vi "HardwareConfiguration.vi"() -> (3 "configured?":bool)   [LabVIEW 2013]
uses:
  InstrControl/InstrumentSetup.vi
  globals/QC_RunInformation.vi
  InstrControl/InstrControl.lvclass
panel:
  in  "Matrix Configurations":bool
  in  "Defaults Multimeter":bool
  in  "Multimeter":enum32{"Keithley 2000"}(tab)
  in  "Range Value\n(0.1 - 100)":dbl=100.0 format="%#.2g"
  in  "Range":u16(ring) items=["Auto", "Manual"]
  in  "Function":u16(ring)=3 items=["AC Current", "DC Current", "AC Voltage", "DC Voltage", "2W-Resistance", "4W-Resistance", "Period", "Frequency", "Temperature", "Diode", "Continuity"]
  in  "Address KE2000":refnum<visa-resource-name>
  in  "Defaults LCR":bool
  in  "LCRs":enum32{"WayneKerr 6440B", "WayneKerr 6425"}(tab)
  in  "AC frequency [Hz]":i32=1000 format="%#.3p"
  in  "RC Configuration":u16(ring) items=["serial", "parallel"]
  in  "AC amplitude [V]":sgl=0.1
  in  "Address WK6440B":refnum<visa-resource-name>
  in  "Address WK6425":refnum<visa-resource-name>
  in  "AC amplitude [V] WK6425":sgl=0.1 caption="AC amplitude [V]"
  in  "RC Configuration WK6425":u16(ring) caption="RC Configuration" items=["serial", "parallel"]
  in  "AC frequency [Hz] WK6425":i32=1000 caption="AC frequency [Hz]" format="%#.3p"
  in  "VISA address":refnum<visa-resource-name>="COM24" caption="Arduino address"
  out "Programm uploaded?":string="Make sure programme is uploaded to Arduino Uno ->"
  in  "Blank Button":bool
  in  "Supplies":T1(tab)
  in  "Front/Rear Output KE2410":u16(ring) caption="Front/Rear Output (not yet implemented)" items=["Front", "Rear"]
  in  "Current Limit [µA] 2410":sgl=100.0 caption="Current Limit [µA]"
  in  "Address KE2410":refnum<visa-resource-name>
  in  "Address KE2410_2":refnum<visa-resource-name>
  in  "Current Limit [µA] 2410_2":sgl=100.0 caption="Current Limit [µA]"
  in  "Front/Rear Output KE2410_2":u16(ring) caption="Front/Rear Output (not yet implemented)" items=["Front", "Rear"]
  in  "Address KE487":refnum<visa-resource-name>
  in  "Compliance":u16(ring) items=["20µA", "2mA"]
  in  "Range:":u16(ring) items=["Autorange", "2nA", "20nA", "200nA", "2 microAmp", "20 microAmp", "200 microAmp", "2 milliAmp"]
  in  "Current Limit 6517":u16(ring)=1 caption="Current Limit" items=["OFF", "ON"]
  in  "Address KE6517":refnum<visa-resource-name>
  in  "Address KE6517_2":refnum<visa-resource-name>
  in  "Current Limit 6517_2":u16(ring)=1 caption="Current Limit" items=["OFF", "ON"]
  in  "current compliance \nlevel [mA]":dbl=0.0001 format="%.4f"
  in  "compliance/measurement\nrange (auto:0)":u16(ring)=6 items=["auto / auto", "1 nA / 1.1 V", "10 nA / 11 V", "100 nA / 110 V", "0.001 mA / 110 V", "0.01 mA / 110 V", "0.1 mA / 110 V", "1 mA / 110 V", "10 mA / 110 V", "100 mA / 110 V"]
  in  "Address KE236":refnum<visa-resource-name>
  in  "Defaults Supply":bool
  in  "OK Button":bool
  # "Hardware Configuration"
  # "Multimeter Configuration"
  # "Supply Configuration"
  # "Arduino Configuration"
  # "LCR Configuration"
  # "(Only for initialisation)"
  # "(Only for initialisation)"
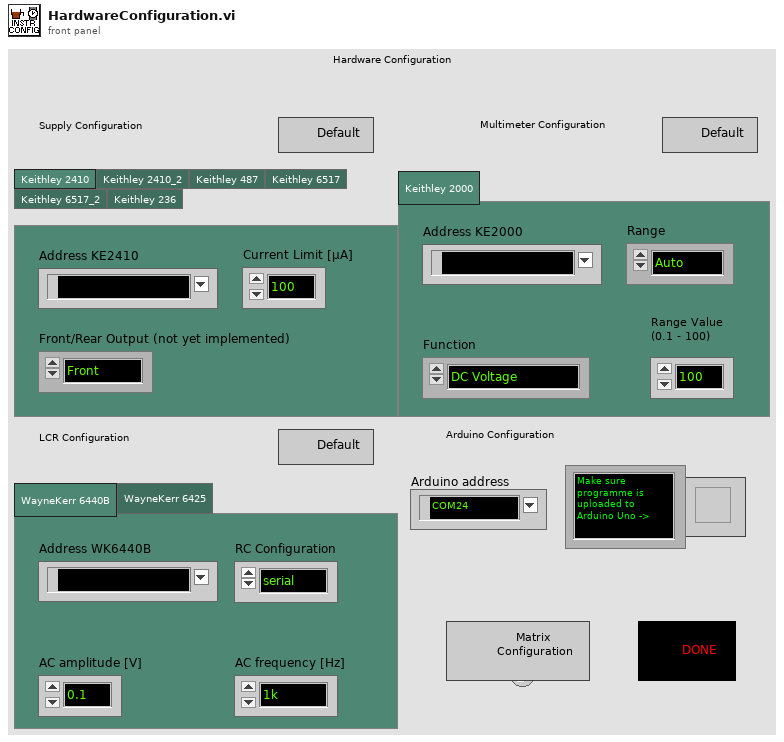
[diagram p1: front panel]
types:
  T1 = enum32{"Keithley 2410", "Keithley 2410_2", "Keithley 487", "Keithley 6517", "Keithley 6517_2", "Keithley 236"}
  T2 = cluster{"KE 2410":cluster{"Instrument name":string, "address":refnum<visa-resource-name>, "Instrument type":u16}, "KE 2410_2":cluster{"Instrument name":string, "address":refnum<visa-resource-name>, "Instrument type":u16}, "KE 6517":cluster{"Instrument name":string, "address":refnum<visa-resource-name>, "Instrument type":u16}, "KE 6517_2":cluster{"Instrument name":string, "address":refnum<visa-resource-name>, "Instrument type":u16}, "KE 487":cluster{"Instrument name":string, "address":refnum<visa-resource-name>, "Instrument type":u16}, "KE 236":cluster{"Instrument name":string, "address":refnum<visa-resource-name>, "Instrument type":u16}, "WK 6440B":cluster{"Instrument name":string, "address":refnum<visa-resource-name>, "Instrument type":u16}, "WK 6425":cluster{"Instrument name":string, "address":refnum<visa-resource-name>, "Instrument type":u16}, "HP 4263B":cluster{"Instrument name":string, "address":refnum<visa-resource-name>, "Instrument type":u16}, "Pickering Matrix":cluster{"Instrument name":string, "address":refnum<visa-resource-name>, "Instrument type":u16}, "KE 2000":cluster{"Instrument name":string, "address":refnum<visa-resource-name>, "Instrument type":u16}, "KE3706A Switching":cluster{"Instrument name":string, "address":refnum<visa-resource-name>, "Instrument type":u16}}
  T3 = cluster{"VISA address":refnum<visa-resource-name>, "T sensor":enum16{"SHT", "DS"}, "Arduino":refnum<class "ArduinoControl.lvclass">}
  T4 = cluster{"Range":u16, "Range Value":dbl, "Function":u16, "KE2000":refnum<class "KE2000.lvclass">}
  T5 = cluster{"Current Limit":sgl, "Front/Rear Output:":u16, "KE2410":refnum<class "KE2410.lvclass">}
  T6 = cluster{"Compliance":u16, "Range:":u16, "KE487":refnum<class "KE487.lvclass">}
  T7 = cluster{"Current Limit":u16, "KE6517":refnum<class "KE6517.lvclass">}
  T8 = cluster{"current \ncompliance level":dbl, "compliance/\nmeasurement range (auto:0)":u16, "KE236":refnum<class "KE236.lvclass">}
  T9 = cluster{"Sensor Serial No.:":string, "Wafer:":string, "Batch:":string, "Manufacturer:":string, "Device Category:":string, "Database Serial No.:":string, "Date Initiated:":string, "Time Initiated:":string, "Test":string, "Probeplan used:":string, "End of Run comment:":string, "User:":string, "Vbias SMU":string, "LCR":string, "Test SMU":string, "Test DMM":string}
  T10 = cluster{"RC Configuration":u16, "AC amplitude [V]":dbl, "AC frequency [Hz]":i32, "WK6440B":refnum<class "WK6440B.lvclass">}
  T11 = cluster{"RC Configuration":u16, "AC amplitude [V]":dbl, "AC frequency [Hz]":i32, "WK6425":refnum<class "WK6425.lvclass">}
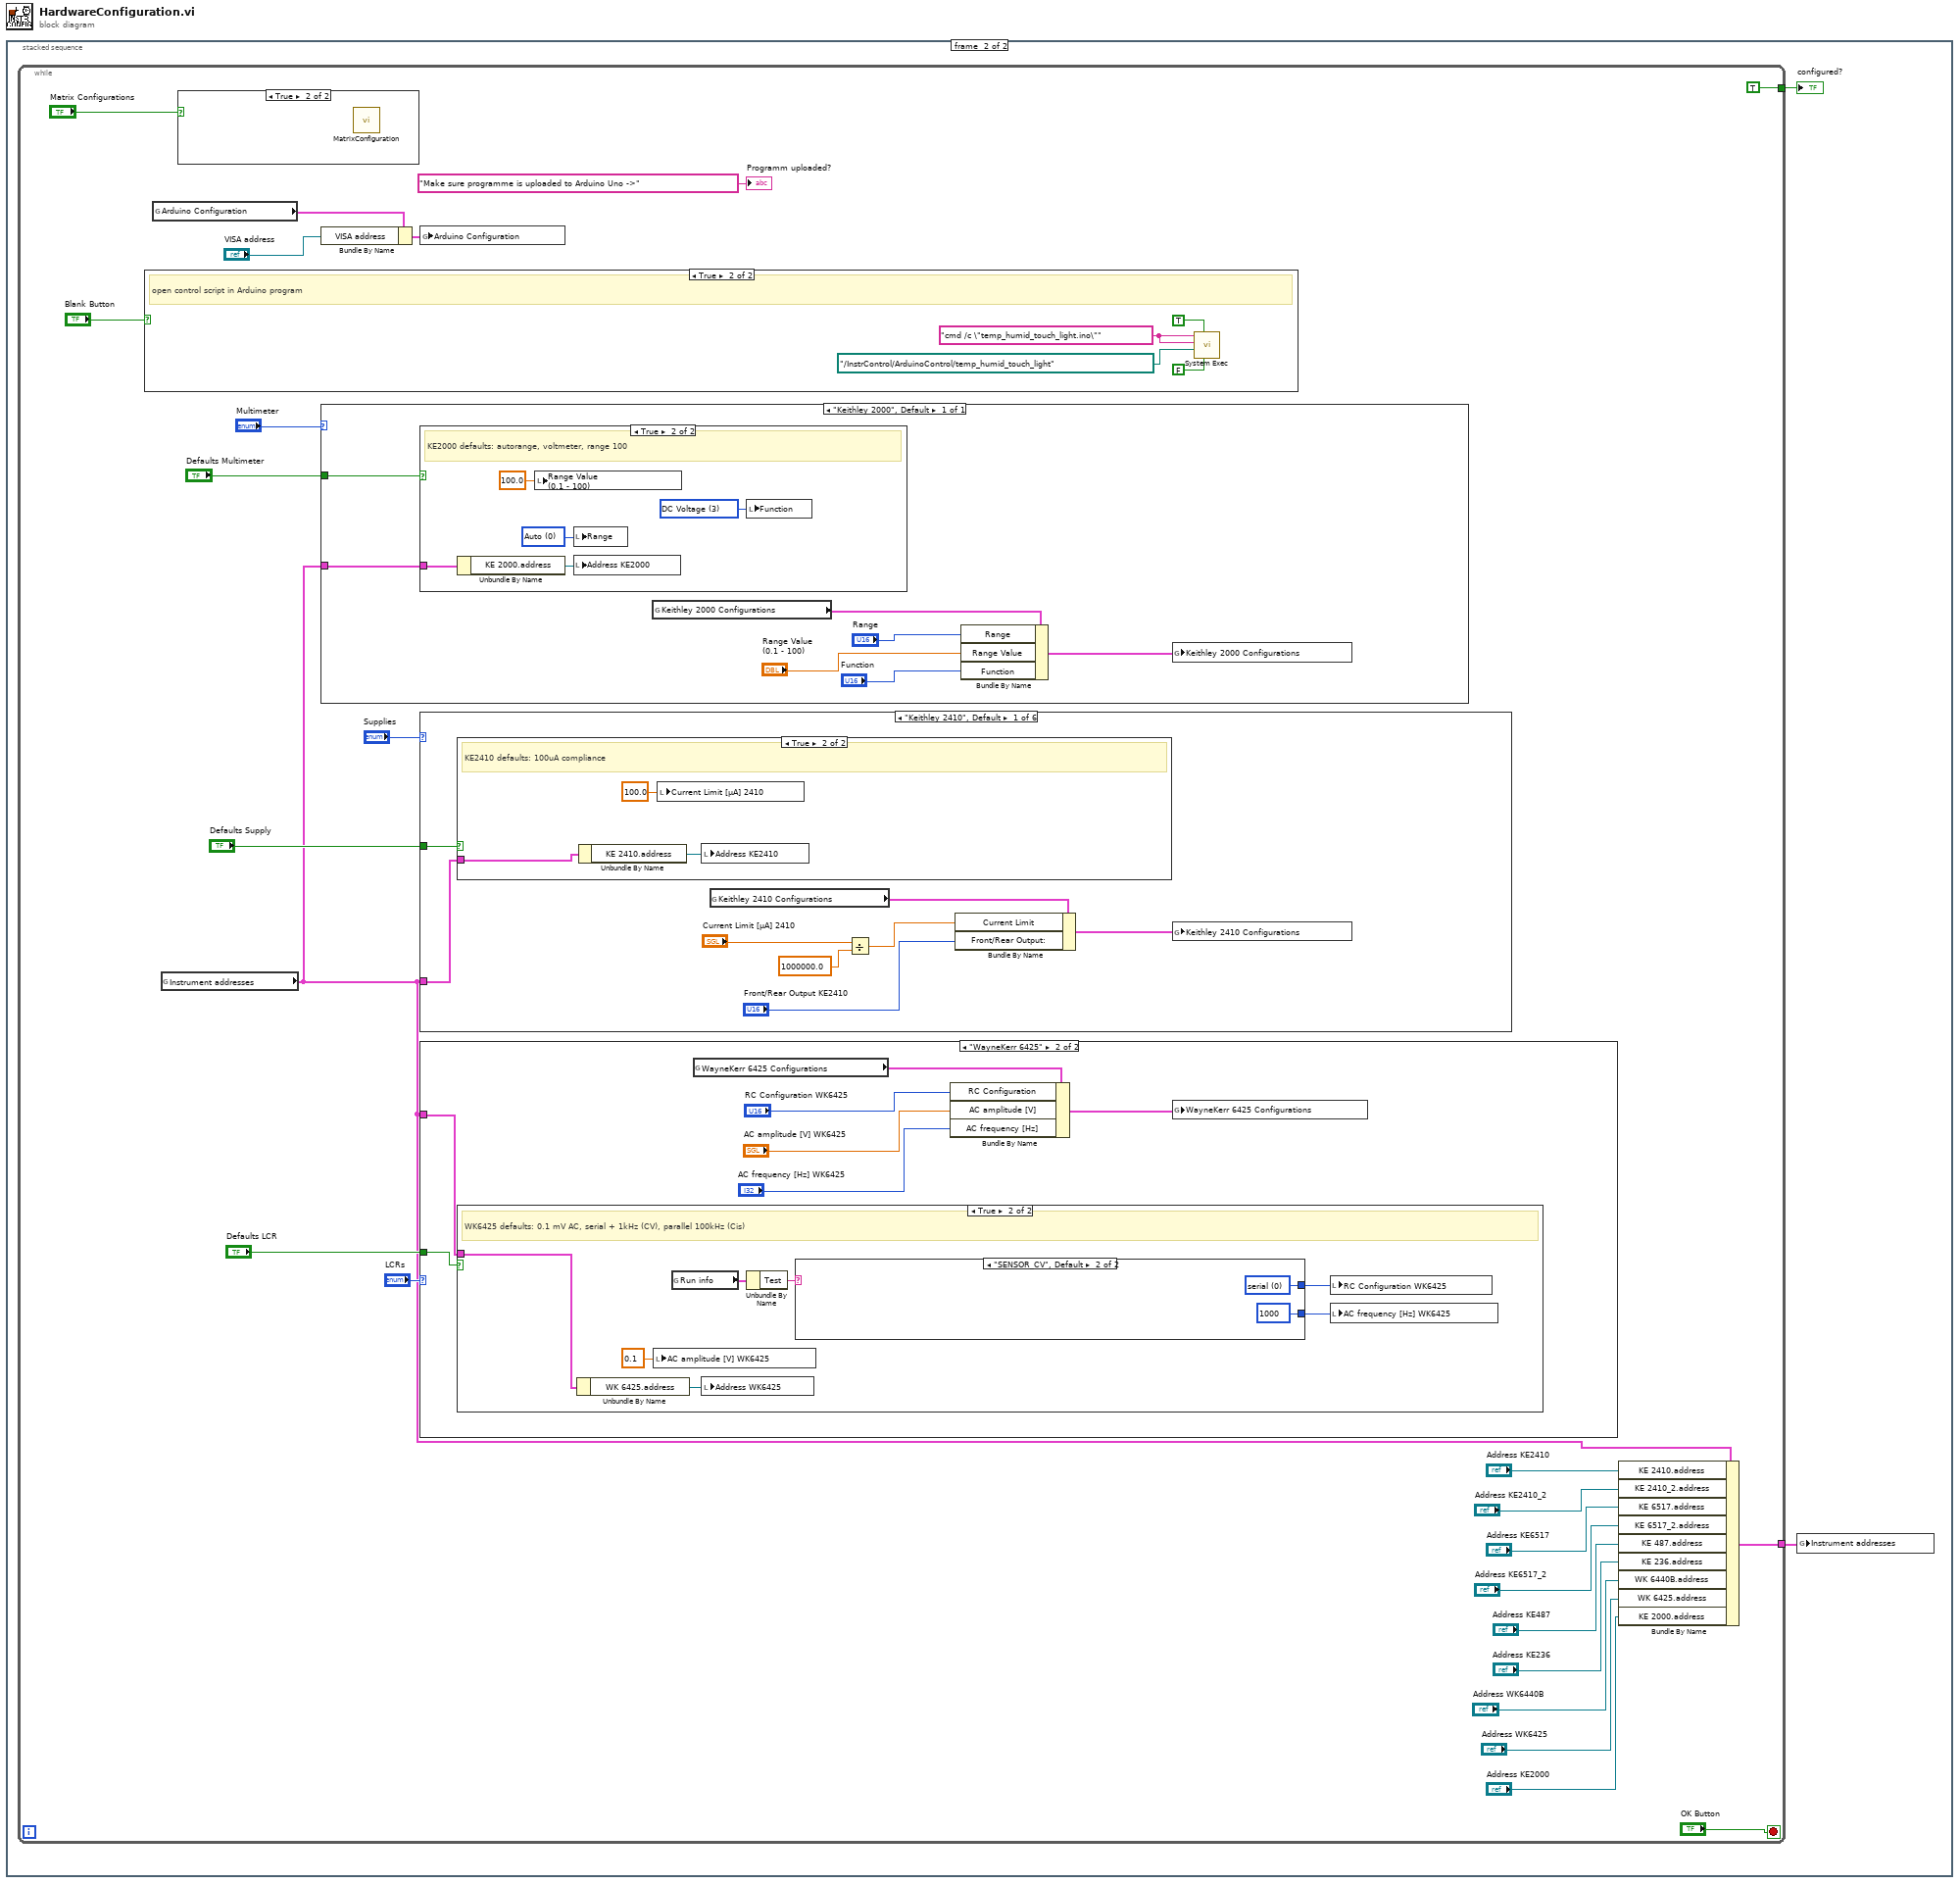
[diagram p0: block diagram]
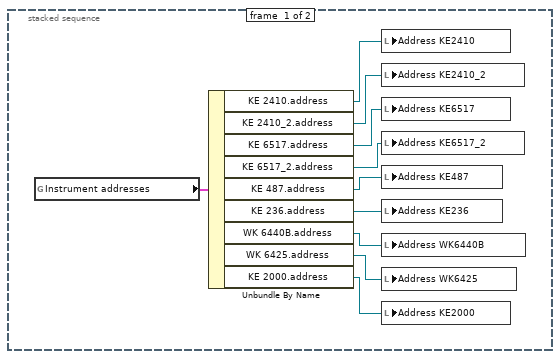
[diagram p2: hidden frame]
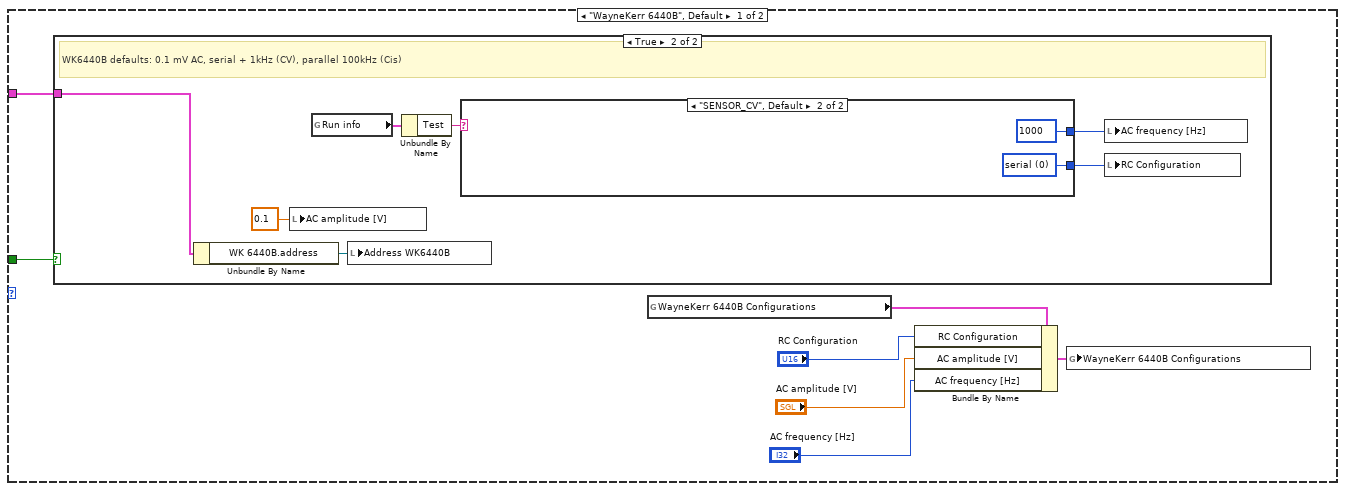
[diagram p6: hidden frame]
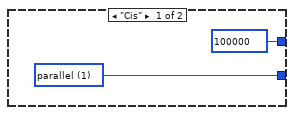
[diagram p8: hidden frame]
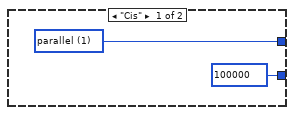
[diagram p10: hidden frame]
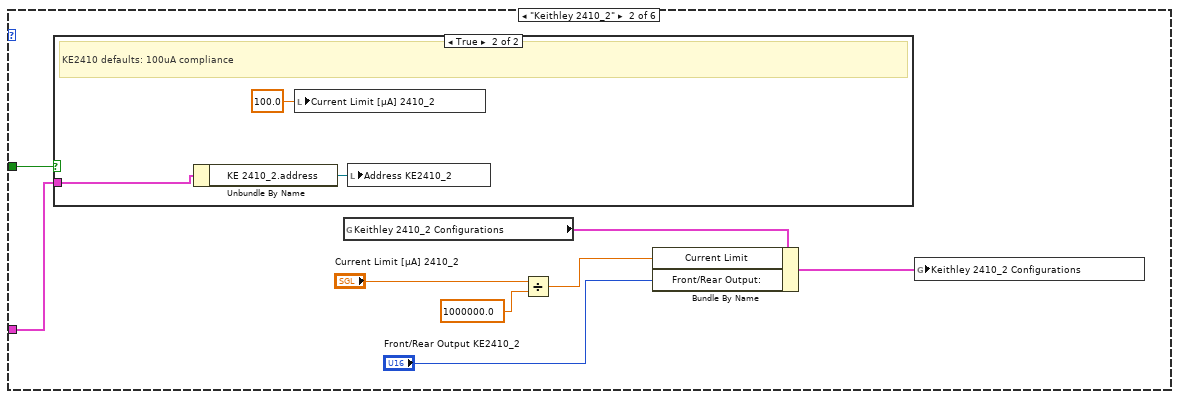
[diagram p12: hidden frame]
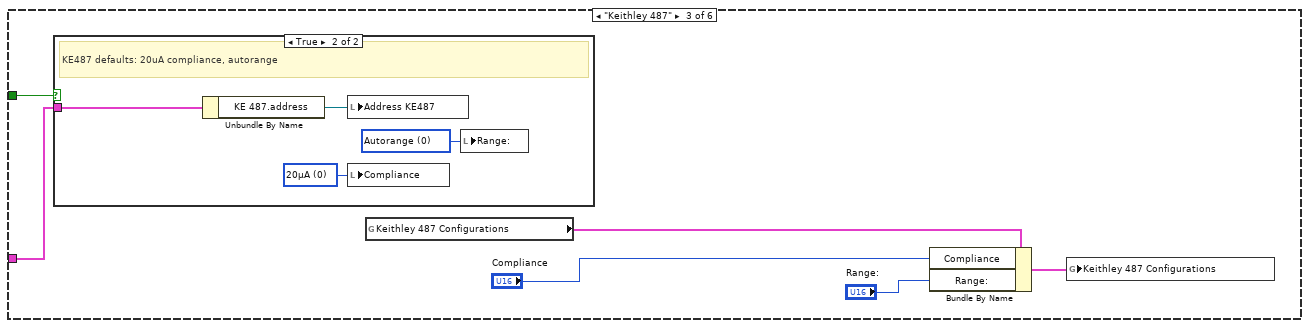
[diagram p14: hidden frame]
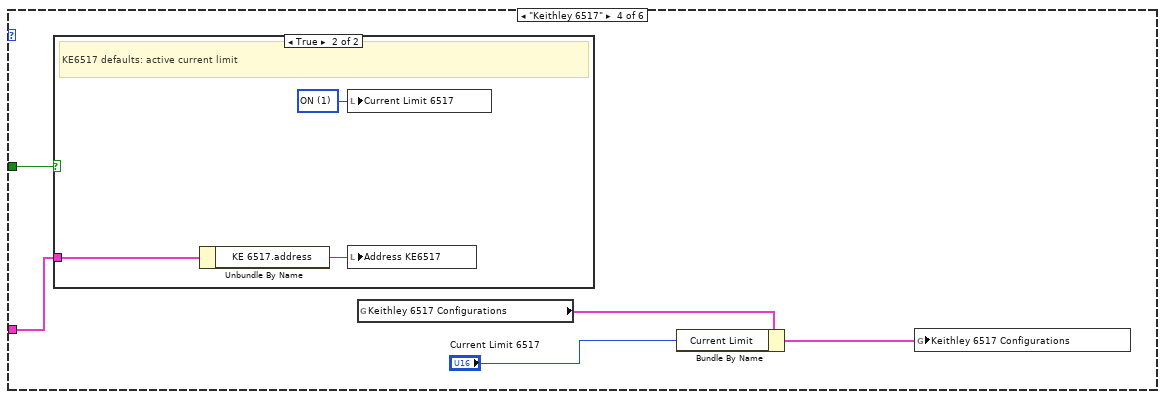
[diagram p16: hidden frame]
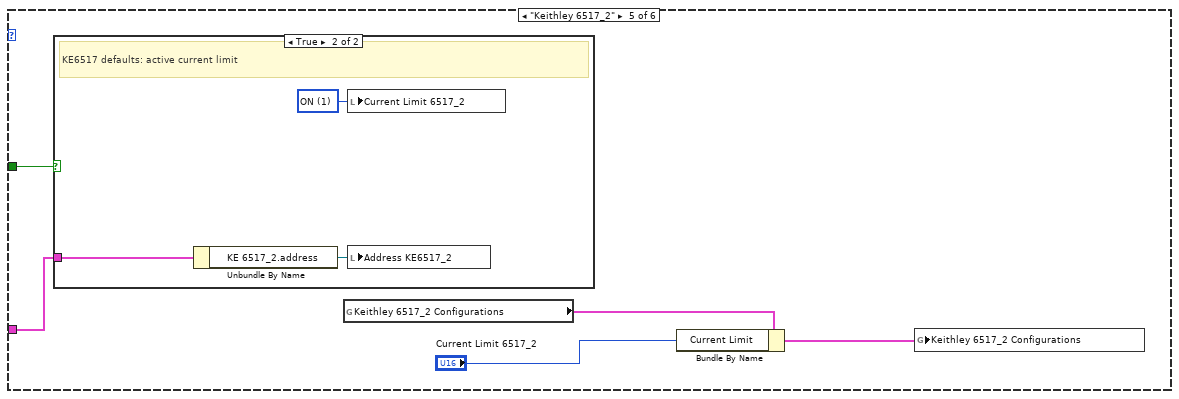
[diagram p18: hidden frame]
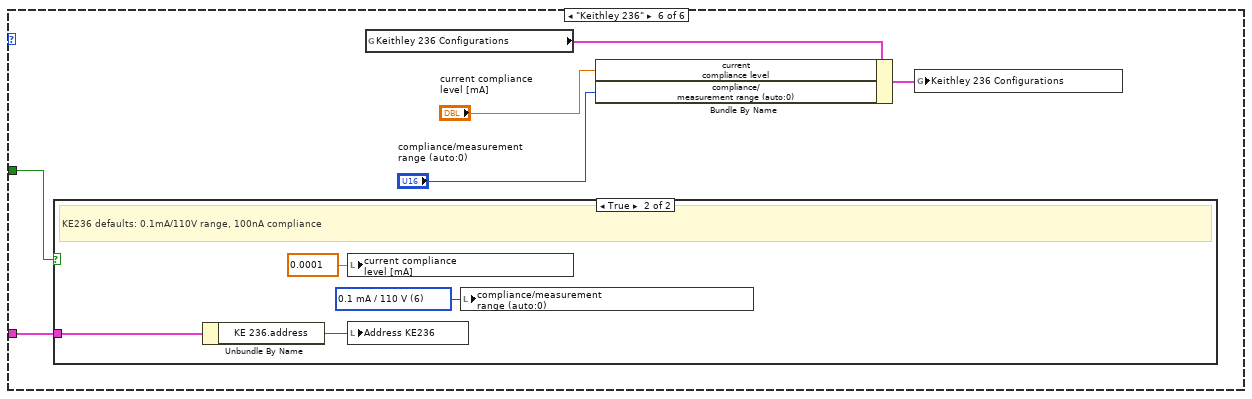
[diagram p20: hidden frame]
diagram:
  n1 = stacked-sequence {
    frame #0 {
      n2 = global read "InstrumentSetup.vi" "Instrument addresses"() -> (w10:T2)
      n3 = Unbundle By Name(w10) -> ("KE 2410.address"=w9:refnum<visa-resource-name>, "KE 2410_2.address"=w2:refnum<visa-resource-name>, "KE 6517.address"=w8:refnum<visa-resource-name>, "KE 6517_2.address"=w1:refnum<visa-resource-name>, "KE 487.address"=w7:refnum<visa-resource-name>, "KE 236.address"=w6:refnum<visa-resource-name>, "WK 6440B.address"=w5:refnum<visa-resource-name>, "WK 6425.address"=w4:refnum<visa-resource-name>, "KE 2000.address"=w3:refnum<visa-resource-name>)
      n4 = local write "Address KE2410"(w9) -> ()
      n5 = local write "Address KE2410_2"(w2) -> ()
      n6 = local write "Address KE6517"(w8) -> ()
      n7 = local write "Address KE6517_2"(w1) -> ()
      n8 = local write "Address KE487"(w7) -> ()
      n9 = local write "Address KE236"(w6) -> ()
      n10 = local write "Address WK6440B"(w5) -> ()
      n11 = local write "Address WK6425"(w4) -> ()
      n12 = local write "Address KE2000"(w3) -> ()
    }
    frame #1 {
      n13 = while {
        tunnel: [TRUE] -> w12
        tunnel: [w21] -> w11
        stop <- "OK Button" stop-if-true
        n14 = case shown="True" "Blank Button" {
          frame False {
          }
          frame True {
            w39 = "cmd /c \"temp_humid_touch_light.ino\""
            # "open control script in Arduino program"
            n15 = call <vilib>:"System Exec.vi"("run minimized? (F)"=FALSE, "wait until completion? (T)"=TRUE, "working directory"=path "../InstrControl/ArduinoControl/temp_humid_touch_light", "standard input"=w39, "command line"=w39) -> ()  [unwired: 3 in, 4 out]
          }
        }
        n16 = global read "InstrumentSetup.vi" "Arduino Configuration"() -> (w28:T3)
        n17 = global read "InstrumentSetup.vi" "Instrument addresses"() -> (w23:T2)
        n18 = case shown="True" "Matrix Configurations" {
          frame False {
          }
          frame True {
            n19 = call "MatrixConfiguration.vi"() -> ()  [unwired: 12 in]
          }
        }
        n20 = Bundle By Name(cluster=w28, "VISA address"="VISA address") -> (w27:T3)
        n21 = case shown="\"Keithley 2000\", Default" "Multimeter" {
          tunnel: "Defaults Multimeter" -> [w48]
          tunnel: w23 -> [w45]
          frame "Keithley 2000", Default {
            n22 = case shown="True" w48 {
              tunnel: w45 -> [_ w53]
              frame False {
              }
              frame True {
                w51 = u16 0 items=["Auto", "Manual"] ("Range")
                w52 = u16 3 items=["AC Current", "DC Current", "AC Voltage", "DC Voltage", "2W-Resistance", "4W-Resistance", "Period", "Frequency", "Temperature", "Diode", "Continuity"] ("Function")
                # "KE2000 defaults: autorange, voltmeter, range 100"
                n23 = Unbundle By Name(w53) -> ("KE 2000.address"=w49:refnum<visa-resource-name>)
                n24 = local write "Range Value\n(0.1 - 100)"(100.0 ("Range Value\n(0.1 - 100)")) -> ()
                n25 = local write "Range"(w51) -> ()
                n26 = local write "Address KE2000"(w49) -> ()
                n27 = local write "Function"(w52) -> ()
              }
            }
            n28 = global read "InstrumentSetup.vi" "Keithley 2000 Configurations"() -> (w47:T4)
            n29 = Bundle By Name(cluster=w47, "Range"="Range", "Range Value"="Range Value\n(0.1 - 100)", "Function"="Function") -> (w46:T4)
            n30 = global write "InstrumentSetup.vi" "Keithley 2000 Configurations"(w46) -> ()
          }
        }
        n31 = global write "InstrumentSetup.vi" "Arduino Configuration"(w27) -> ()
        n32 = case shown="\"Keithley 2410\", Default" "Supplies" {
          tunnel: "Defaults Supply" -> [w97 w102 w117 w126 w133 w143]
          tunnel: w23 -> [w92 w103 w114 w123 w134 w140]
          frame "Keithley 2410", Default {
            n33 = case shown="True" w97 {
              tunnel: w92 -> [_ w100]
              frame False {
              }
              frame True {
                # "KE2410 defaults: 100uA compliance"
                n34 = Unbundle By Name(w100) -> ("KE 2410.address"=w98:refnum<visa-resource-name>)
                n35 = local write "Current Limit [µA] 2410"(100.0) -> ()
                n36 = local write "Address KE2410"(w98) -> ()
              }
            }
            n37 = global read "InstrumentSetup.vi" "Keithley 2410 Configurations"() -> (w96:T5)
            n38 = Divide(x="Current Limit [µA] 2410", y=1000000.0) -> (x/y=w93:dbl)
            n39 = Bundle By Name(cluster=w96, "Current Limit"=w93, "Front/Rear Output:"="Front/Rear Output KE2410") -> (w95:T5)
            n40 = global write "InstrumentSetup.vi" "Keithley 2410 Configurations"(w95) -> ()
          }
          frame "Keithley 2410_2" {
            n41 = case shown="True" w102 {
              tunnel: w103 -> [_ w111]
              frame False {
              }
              frame True {
                # "KE2410 defaults: 100uA compliance"
                n42 = Unbundle By Name(w111) -> ("KE 2410_2.address"=w109:refnum<visa-resource-name>)
                n43 = local write "Current Limit [µA] 2410_2"(100.0) -> ()
                n44 = local write "Address KE2410_2"(w109) -> ()
              }
            }
            n45 = global read "InstrumentSetup.vi" "Keithley 2410_2 Configurations"() -> (w104:T5)
            n46 = Divide(x="Current Limit [µA] 2410_2", y=1000000.0) -> (x/y=w106:dbl)
            n47 = Bundle By Name(cluster=w104, "Current Limit"=w106, "Front/Rear Output:"="Front/Rear Output KE2410_2") -> (w105:T5)
            n48 = global write "InstrumentSetup.vi" "Keithley 2410_2 Configurations"(w105) -> ()
          }
          frame "Keithley 487" {
            n49 = case shown="True" w117 {
              tunnel: w114 -> [_ w121]
              frame False {
              }
              frame True {
                w119 = u16 0 items=["Autorange", "2nA", "20nA", "200nA", "2 microAmp", "20 microAmp", "200 microAmp", "2 milliAmp"] ("Range:")
                w120 = u16 0 items=["20µA", "2mA"] ("Compliance")
                # "KE487 defaults: 20uA compliance, autorange"
                n50 = Unbundle By Name(w121) -> ("KE 487.address"=w118:refnum<visa-resource-name>)
                n51 = local write "Address KE487"(w118) -> ()
                n52 = local write "Compliance"(w120) -> ()
                n53 = local write "Range:"(w119) -> ()
              }
            }
            n54 = global read "InstrumentSetup.vi" "Keithley 487 Configurations"() -> (w116:T6)
            n55 = Bundle By Name(cluster=w116, "Compliance"="Compliance", "Range:"="Range:") -> (w115:T6)
            n56 = global write "InstrumentSetup.vi" "Keithley 487 Configurations"(w115) -> ()
          }
          frame "Keithley 6517" {
            n57 = case shown="True" w126 {
              tunnel: w123 -> [_ w129]
              frame False {
              }
              frame True {
                w128 = u16 1 items=["OFF", "ON"] ("Current Limit")
                # "KE6517 defaults: active current limit"
                n58 = Unbundle By Name(w129) -> ("KE 6517.address"=w127:refnum<visa-resource-name>)
                n59 = local write "Current Limit 6517"(w128) -> ()
                n60 = local write "Address KE6517"(w127) -> ()
              }
            }
            n61 = global read "InstrumentSetup.vi" "Keithley 6517 Configurations"() -> (w125:T7)
            n62 = Bundle By Name(cluster=w125, "Current Limit"="Current Limit 6517") -> (w124:T7)
            n63 = global write "InstrumentSetup.vi" "Keithley 6517 Configurations"(w124) -> ()
          }
          frame "Keithley 6517_2" {
            n64 = case shown="True" w133 {
              tunnel: w134 -> [_ w137]
              frame False {
              }
              frame True {
                w136 = u16 1 items=["OFF", "ON"] ("Current Limit")
                # "KE6517 defaults: active current limit"
                n65 = Unbundle By Name(w137) -> ("KE 6517_2.address"=w135:refnum<visa-resource-name>)
                n66 = local write "Current Limit 6517_2"(w136) -> ()
                n67 = local write "Address KE6517_2"(w135) -> ()
              }
            }
            n68 = global read "InstrumentSetup.vi" "Keithley 6517_2 Configurations"() -> (w132:T7)
            n69 = Bundle By Name(cluster=w132, "Current Limit"="Current Limit 6517_2") -> (w131:T7)
            n70 = global write "InstrumentSetup.vi" "Keithley 6517_2 Configurations"(w131) -> ()
          }
          frame "Keithley 236" {
            n71 = case shown="True" w143 {
              tunnel: w140 -> [_ w147]
              frame False {
              }
              frame True {
                w145 = u16 6 items=["auto / auto", "1 nA / 1.1 V", "10 nA / 11 V", "100 nA / 110 V", "0.001 mA / 110 V", "0.01 mA / 110 V", "0.1 mA / 110 V", "1 mA / 110 V", "10 mA / 110 V", "100 mA / 110 V"] ("compliance/\nmeasurement range (auto:0)")
                # "KE236 defaults: 0.1mA/110V range, 100nA compliance"
                n72 = Unbundle By Name(w147) -> ("KE 236.address"=w144:refnum<visa-resource-name>)
                n73 = local write "current compliance \nlevel [mA]"(0.0001 ("current \ncompliance level")) -> ()
                n74 = local write "Address KE236"(w144) -> ()
                n75 = local write "compliance/measurement\nrange (auto:0)"(w145) -> ()
              }
            }
            n76 = global read "InstrumentSetup.vi" "Keithley 236 Configurations"() -> (w141:T8)
            n77 = Bundle By Name(cluster=w141, "current \ncompliance level"="current compliance \nlevel [mA]", "compliance/\nmeasurement range (auto:0)"="compliance/measurement\nrange (auto:0)") -> (w142:T8)
            n78 = global write "InstrumentSetup.vi" "Keithley 236 Configurations"(w142) -> ()
          }
        }
        n79 = case shown="\"WayneKerr 6425\"" "LCRs" {
          tunnel: "Defaults LCR" -> [w58 w76]
          tunnel: w23 -> [w57 w75]
          frame "WayneKerr 6440B", Default {
            n80 = case shown="True" w58 {
              tunnel: w57 -> [_ w67]
              frame False {
              }
              frame True {
                # "WK6440B defaults: 0.1 mV AC, serial + 1kHz (CV), parallel 100kHz (Cis)"
                n81 = Unbundle By Name(w67) -> ("WK 6440B.address"=w61:refnum<visa-resource-name>)
                n82 = local write "AC amplitude [V]"(0.1) -> ()
                n83 = global read "QC_RunInformation.vi" "Run info"() -> (w63:T9)
                n84 = local write "Address WK6440B"(w61) -> ()
                n85 = Unbundle By Name(w63) -> ("Test"=w62:string)
                n86 = case shown="\"SENSOR_CV\", Default" w62 {
                  tunnel: [w69 w71] -> w65
                  tunnel: [100000 1000] -> w64
                  frame "Cis" {
                    w69 = u16 1 items=["serial", "parallel"] ("RC Configuration")
                  }
                  frame "SENSOR_CV", Default {
                    w71 = u16 0 items=["serial", "parallel"] ("RC Configuration")
                  }
                }
                n87 = local write "AC frequency [Hz]"(w64) -> ()
                n88 = local write "RC Configuration"(w65) -> ()
              }
            }
            n89 = global read "InstrumentSetup.vi" "WayneKerr 6440B Configurations"() -> (w60:T10)
            n90 = Bundle By Name(cluster=w60, "RC Configuration"="RC Configuration", "AC amplitude [V]"="AC amplitude [V]", "AC frequency [Hz]"="AC frequency [Hz]") -> (w59:T10)
            n91 = global write "InstrumentSetup.vi" "WayneKerr 6440B Configurations"(w59) -> ()
          }
          frame "WayneKerr 6425" {
            n92 = case shown="True" w76 {
              tunnel: w75 -> [_ w85]
              frame False {
              }
              frame True {
                # "WK6425 defaults: 0.1 mV AC, serial + 1kHz (CV), parallel 100kHz (Cis)"
                n93 = Unbundle By Name(w85) -> ("WK 6425.address"=w79:refnum<visa-resource-name>)
                n94 = local write "AC amplitude [V] WK6425"(0.1) -> ()
                n95 = global read "QC_RunInformation.vi" "Run info"() -> (w81:T9)
                n96 = local write "Address WK6425"(w79) -> ()
                n97 = Unbundle By Name(w81) -> ("Test"=w80:string)
                n98 = case shown="\"SENSOR_CV\", Default" w80 {
                  tunnel: [w87 w89] -> w83
                  tunnel: [100000 1000] -> w82
                  frame "Cis" {
                    w87 = u16 1 items=["serial", "parallel"] ("RC Configuration")
                  }
                  frame "SENSOR_CV", Default {
                    w89 = u16 0 items=["serial", "parallel"] ("RC Configuration")
                  }
                }
                n99 = local write "RC Configuration WK6425"(w83) -> ()
                n100 = local write "AC frequency [Hz] WK6425"(w82) -> ()
              }
            }
            n101 = global read "InstrumentSetup.vi" "WayneKerr 6425 Configurations"() -> (w78:T11)
            n102 = Bundle By Name(cluster=w78, "RC Configuration"="RC Configuration WK6425", "AC amplitude [V]"="AC amplitude [V] WK6425", "AC frequency [Hz]"="AC frequency [Hz] WK6425") -> (w77:T11)
            n103 = global write "InstrumentSetup.vi" "WayneKerr 6425 Configurations"(w77) -> ()
          }
        }
        n104 = Bundle By Name(cluster=w23, "KE 2410.address"="Address KE2410", "KE 2410_2.address"="Address KE2410_2", "KE 6517.address"="Address KE6517", "KE 6517_2.address"="Address KE6517_2", "KE 487.address"="Address KE487", "KE 236.address"="Address KE236", "WK 6440B.address"="Address WK6440B", "WK 6425.address"="Address WK6425", "KE 2000.address"="Address KE2000") -> (w21:T2)
        "Programm uploaded?" <- "Make sure programme is uploaded to Arduino Uno ->"
      }
      "configured?" <- w12
      n105 = global write "InstrumentSetup.vi" "Instrument addresses"(w11) -> ()
    }
  }
